vi "Query ViString.vi"(8 "error in (no error)":errorcluster, 10 "Query":string, 11 "VISA resource name":refnum<visa-resource-name>) -> (0 "error out":errorcluster, 2 "Response Value":string, 3 "VISA resource name out":refnum<visa-resource-name>)   [LabVIEW 2015, in "Rohde&Schwarz CMXP Base.lvlib"]
doc: "This VI sends the SCPI query to the instrument, and reads the response. The response is trimmed of leading and trailing white characters (\\n, \\r, \\t, \\s).\nThe length of the response is not limited. If it is longer than 65kB, the transfer is performed over VISA interface in 65kB bytes long chunks and combined together.\nDo not use this VI if you expect binary data response (data starting with # character) e.g. file data content or trace data. For that purpose use <b>Read To File From Instrument.vi</b> or more general <b>Bin Data To File From Instrument.vi</b>"
uses:
  <instrlib>/Rohde&Schwarz CMXP Base/Rohde&Schwarz CMXP Base.lvlib
  <instrlib>/Rohde&Schwarz CMXP Base/Private/rsidr_core.llb/rsidr_core.lvlib
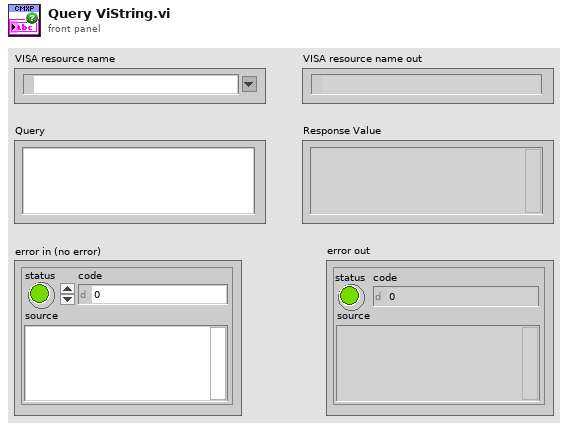
[diagram p1: front panel]
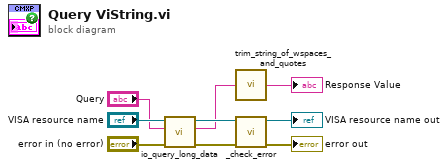
[diagram p0: block diagram]
diagram:
  n1 = call <instrlib>:"io_query_long_data.vi"("error in"="error in (no error)", "write buffer"="Query", "VISA resource name"="VISA resource name") -> ("error out"=w7:errorcluster, "read buffer"=w1:string, "VISA resource name out"=w6:refnum<visa-resource-name>)  [unwired: 6 in]
  n2 = call <instrlib>:"trim_string_of_wspaces_and_quotes.vi"("String in"=w1) -> ("String out"=→"Response Value":string)  [unwired: 4 in]
  n3 = call <instrlib>:"_check_error.vi"("error in (no error)"=w7, "VISA resource name"=w6) -> ("error out"=→"error out":errorcluster, "VISA resource name out"=→"VISA resource name out":refnum<visa-resource-name>)  [unwired: 8 in]
